vi "Write Com_Set.vi"(8 "error in (no error)":errorcluster, 10 "Com_Set":T1, 11 "RS232 In":refnum<class "RS232.lvclass">) -> (0 "error out":errorcluster, 3 "RS232 Out":refnum<class "RS232.lvclass">)   [LabVIEW 2019, in "RS232.lvclass"]
uses:
  RS232.lvclass
  SettingCtrl.ctl
  RS232.lvclass/RS232.ctl
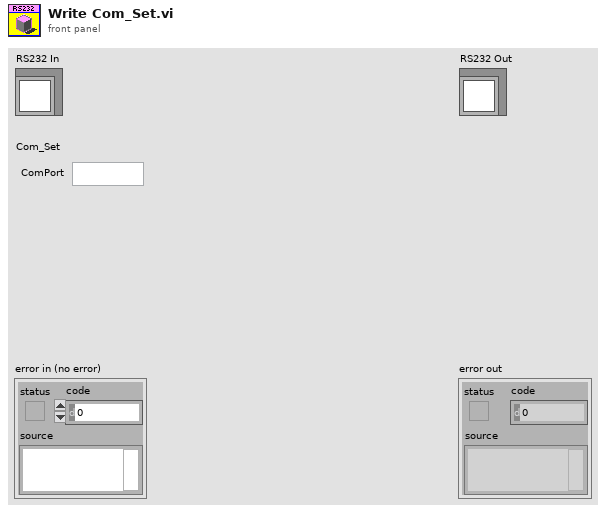
[diagram p1: front panel]
types:
  T1 = typedef "RS232.lvclass/SettingCtrl.ctl" = cluster{"ComPort":string}
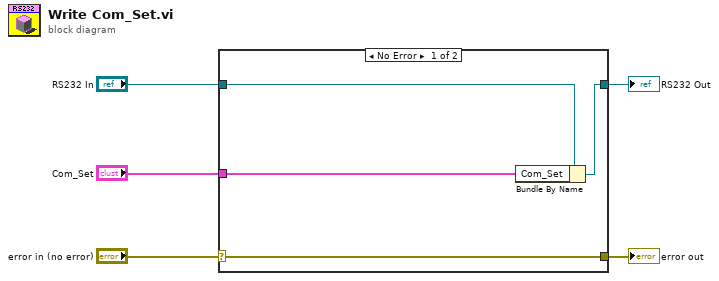
[diagram p0: block diagram]
diagram:
  n1 = case shown="No Error" "error in (no error)" {
    selector: "error in (no error)" -> [w9 w10]
    tunnel: [w9 w10] -> w4
    tunnel: [w7 w11] -> w2
    tunnel: "RS232 In" -> [w8 w11]
    tunnel: "Com_Set" -> [w6 _]
    frame No Error {
      n2 = Bundle By Name(cluster=w8, "Com_Set"=w6) -> (w7:refnum<class "RS232.lvclass">)
    }
    frame Error {
    }
  }
  "error out" <- w4
  "RS232 Out" <- w2
